vi "BT_debugging.vi"() -> ()   [LabVIEW 2016]
panel:
  out "after substring":string
  out "offset past match":i32=5
  out "status":bool
  in  "error out":errorcluster
  out "substring":string
  out "String 2":string
  in  "Pkt Offset":i32=6
  in  "String":string
  # "7"
  # "0A 0B 0C S1 S2"
  # "3345 0A0B 0C84 0181 8701 0000 AC10 524B 0002 FC01 C23C 00F9 D001 C240 00FB AF09 DB48 00F2 8406 2D44 0001 2A17 383F 00FF 13FB 3F3F 0018 6614 8C45 0004 8418 0F43 001C 0107 7D3C 0019 C010 4E31 000E A60F B73A 0017 9409 8B32 00FD A202 5544 0007 7BFC 5A34 0001 0402 1A4D 000B 46F6 1648 0004 0108 8A45 001C 3500 F933 001B 7609 FB39 0021 77FF E736 001E 6706 3F38 0021 250C A238 001A 3EFC 8D3F 000D A80C F442 00FA 3A07 BE42 000B 0801 7D34 00F5 CDFF CC3A 00F3 7FFB 5735 00F3 870E 3138 00FC 8B00 59A5 00EB BEFB DE39 0000 FA02 A148 000C 1FFA 3938 00EE 80F5 7539 0011 03FC 0837 0008 54FA DF3C 0007 0CFE 5C3D 0018 6906 EB3D 0019 CEFF B535 0019 2104 ED4C 000D 04FB C137 0008 6EF6 0F3C 0009 5BF4 3844 0005 3DF5 8837 0007 A1E9 C844 00F7 B6F1 0041 00FA 40E9 D843 0011 DCFF E439 0018 6407 6042 0013 FD02 EE34 001F 6500 7841 0020 4AFB AB37 0018 44D8 5735 000C 9FFD 4744 00F9 7B00 484C 001B 86F7 E64E 0012 41EE 8E3F 001B FAE1 9948 0004 0BE4 09AE 0002 B619 5BA6 000C 14FF 9B40 0010 17F0 EC3F 0010 6AE7 EA48"
  # "3E\n×Üÿÿÿÿÿy¶;úÂ?ü«\tÎFó¸Bëd>ÿÂûË>%D;YCcÁ;1[0Â¬8j\tu0þ$]Cü3ELLölGF~C«\t2Ø\t¹7 5¡X6 \nv6_üR>\naAú*A\n³3ÿÿÿÿÿóüû3óÿ\nê7ürW¨ìJü8&¾GÝú7ïõÛ7üH6û:Õþ];Ç¦;Oÿi4¸´JÿÿÿÿÿöV;\t\"ôBþõê5kêrC÷ññ?úrêsBfÿ¼8á#@tÅ3¢}@ûÍ5ÎÙF4XýCù¤KÑ÷ÂMÂîÍ=;â1GÚä¥°È¨ÃÿÂ?¶ñM>8èG"
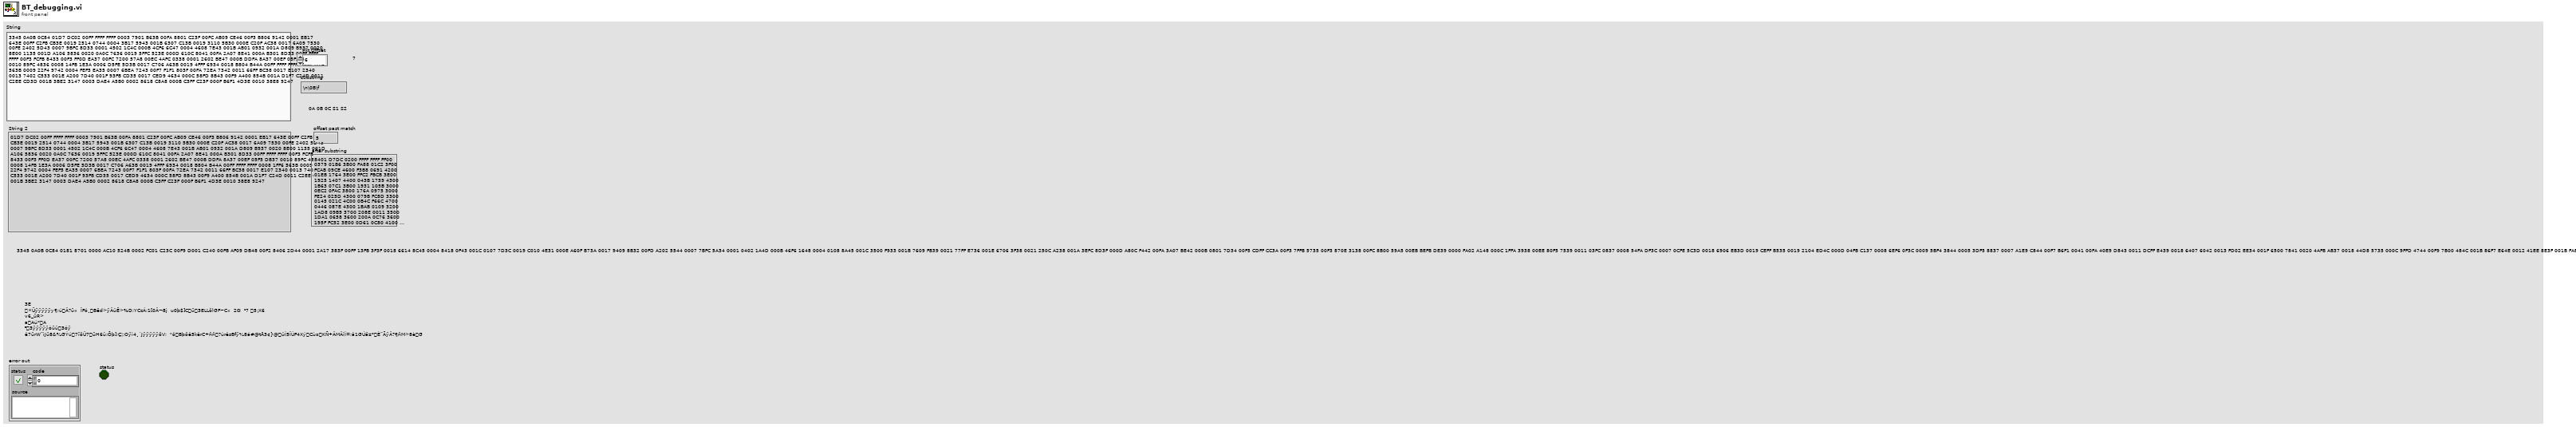
[diagram p1: front panel]
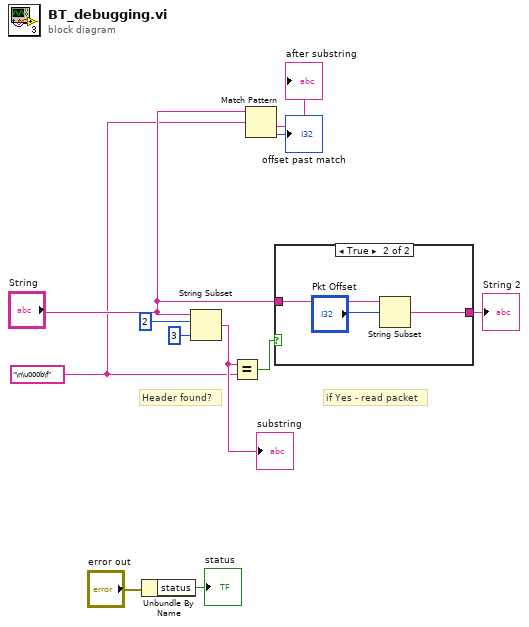
[diagram p0: block diagram]
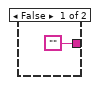
[diagram p2: hidden frame]
diagram:
  w3 = "\n\u000b\f" ("y")
  # "if Yes - read packet"
  # "Header found?"
  n1 = Unbundle By Name("error out") -> ("status"=→"status":bool)
  n2 = String Subset(string="String", offset (0)=2, length (rest)=3 ("length (rest)")) -> (substring=w10:string)
  "substring" <- w10
  n3 = Equal?(x=w10, y=w3) -> (x = y?=w9:bool)
  n4 = Match Pattern(string="String", regular expression=w3) -> (after substring=→"after substring":string, offset past match=→"offset past match":i32)  [unwired: 1 in, 2 out]
  n5 = case shown="True" w9 {
    tunnel: ["" w15] -> w7
    tunnel: "String" -> [_ w14]
    frame False {
    }
    frame True {
      n6 = String Subset(string=w14, offset (0)="Pkt Offset") -> (substring=w15:string)  [unwired: 1 in]
    }
  }
  "String 2" <- w7
